vi "Configure Interval Trigger.vi"(0 "VISA resource name":refnum<visa-resource-name>, 1 "Trigger Slope (0: Rising)":u16(ring) items=["Rising", "Falling"], 2 "Trigger Source (0: Channel 1)":u16(ring) items=["Channel 1", "Channel 2", "Channel 3", "Channel 4", "External", "Pattern", "Ext", "Ext10"], 5 "Trigger Level (0.0 V)":dbl, 9 "Mode (0: Less Than)":u16(ring) items=["Less Than", "Greater Than", "In Range/Out Of Range"], 11 "error in (no error)":errorcluster, 12 "Limit 1 (4 ns)":dbl=4e-09, 13 "Limit 2 (6 ns)":dbl=6e-09) -> (4 "VISA resource name out":refnum<visa-resource-name>, 15 "error out":errorcluster)   [LabVIEW 2018, in "LeCroy Wave Series.lvlib"]
doc: "Configures interval trigger settings. Interval trigger performs over the width of an interval the signal duration (the period) separating two consecutive edges of the same polarity: positive to positive or negative to negative. Use interval trigger to capture intervals that fall short of, or exceed, a given time limit. In addition, you can define a width range to capture any interval that is itself inside or outside the specified range an Exclusion trigger by interval.\n\nNote: \"External\" is included for the purpose of backwards compatibility. Use EXT or EXT10 for best results."
uses:
  LeCroy Wave Series.lvlib
panel:
  # "Note: \"External\" is included for the purpose\nof backwards compatibility.  Use EXT or EXT10\nfor best results."
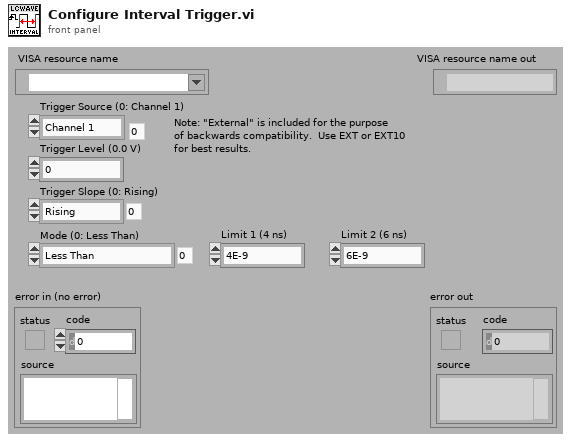
[diagram p1: front panel]
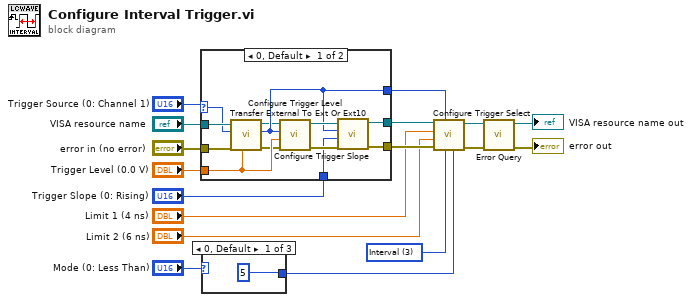
[diagram p0: block diagram]
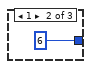
[diagram p2: hidden frame]
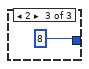
[diagram p3: hidden frame]
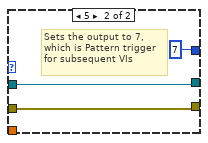
[diagram p4: hidden frame]
diagram:
  w2 = u16 3 items=["Edge", "Dropout", "Glitch", "Interval", "Std", "Sng", "State Qualify", "Edge Qualify"] ("Trigger type")
  n1 = case shown="0, Default" "Trigger Source (0: Channel 1)" {
    selector: "Trigger Source (0: Channel 1)" -> [w21 _]
    tunnel: "VISA resource name" -> [w23 w32]
    tunnel: "error in (no error)" -> [w22 w31]
    tunnel: "Trigger Slope (0: Rising)" -> [w27 _]
    tunnel: [w26 w32] -> w14
    tunnel: [w25 w31] -> w13
    tunnel: "Trigger Level (0.0 V)" -> [w20 _]
    tunnel: [w24 7] -> w1
    frame 0, Default {
      n2 = call "Transfer External To Ext Or Ext10.vi"("Trigger Level"=w20, "error in (no error)"=w22, "Trigger Source With External"=w21, "VISA resource name"=w23) -> ("error out"=w18:errorcluster, "Trigger Source With Ext/Ext10"=w24:u16, "VISA resource name out"=w19:refnum<visa-resource-name>)  [unwired: 5 in]
      n3 = call "Configure Trigger Level.vi"("error in (no error)"=w18, "Trigger Level 1 (0.0 V)"=w20, "Channel (0: Channel 1)"=w24, "VISA resource name"=w19) -> ("error out"=w28:errorcluster, "VISA resource name out"=w29:refnum<visa-resource-name>)  [unwired: 6 in]
      n4 = call "Configure Trigger Slope.vi"("error in (no error)"=w28, "Trigger Slope (0: Rising)"=w27, "Channel (0: Channel 1)"=w24, "VISA resource name"=w29) -> ("error out"=w25:errorcluster, "VISA resource name out"=w26:refnum<visa-resource-name>)  [unwired: 6 in]
    }
    frame 5 {
      # "Sets the output to 7,\nwhich is Pattern trigger\nfor subsequent VIs"
    }
  }
  n5 = case shown="0, Default" "Mode (0: Less Than)" {
    tunnel: [5 6 8] -> w9
    frame 0, Default {
    }
    frame 1 {
    }
    frame 2 {
    }
  }
  n6 = call "Configure Trigger Select.vi"("Hold Type (0: TI)"=w9, "Trigger type"=w2, "Trigger Source (0: Channel 1)"=w1, "error in (no error)"=w13, "Hold Value 2 (6 ns)"="Limit 2 (6 ns)", "Hold Value 1 (4 ns)"="Limit 1 (4 ns)", "VISA resource name"=w14) -> ("error out"=w5:errorcluster, "VISA resource name out"=w6:refnum<visa-resource-name>)  [unwired: 3 in]
  n7 = call "Error Query.vi"("error in (no error)"=w5, "VISA resource name"=w6) -> ("error out"=→"error out":errorcluster, "VISA resource name out"=→"VISA resource name out":refnum<visa-resource-name>)  [unwired: 6 in, 2 out]
